vi "Get Charact Result File Name.vi"(0 "Port1":string, 5 "Port2":string, 9 "Charact Type":string, 11 "error in (no error)":errorcluster) -> (4 "Charact result file name":string, 15 "error out":errorcluster)   [LabVIEW 2023, in "RFFixtureCharact.RFPM.lvlib" / "Charact Result Accessor.lvclass"]
uses:
  Charact Result Accessor.lvclass
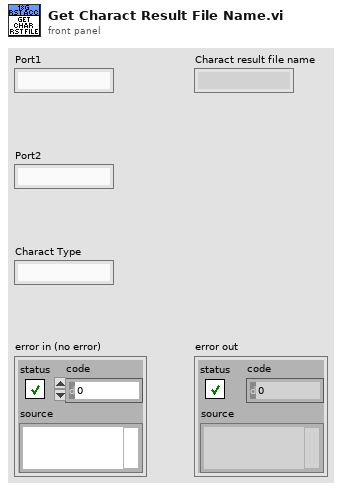
[diagram p1: front panel]
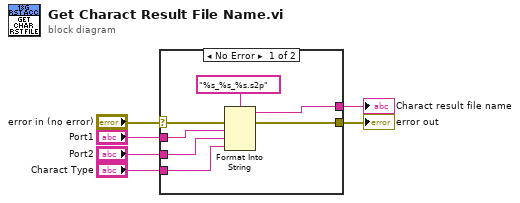
[diagram p0: block diagram]
diagram:
  n1 = case shown="No Error" "error in (no error)" {
    selector: "error in (no error)" -> [w10 w14]
    tunnel: [w12 w14] -> w5
    tunnel: [w11 _] -> w4
    tunnel: "Port1" -> [w9 _]
    tunnel: "Port2" -> [w8 _]
    tunnel: "Charact Type" -> [w7 _]
    frame No Error {
      n2 = Format Into String(format string="%s_%s_%s.s2p", error in=w10, w9, w8, w7) -> (resulting string=w11:string, error out=w12:errorcluster)  [unwired: 1 in]
    }
    frame Error {
    }
  }
  "error out" <- w5
  "Charact result file name" <- w4
